vi "Actor Core.vi"(8 "error in":errorcluster, 11 "Test Actor in":refnum<class "Dummy Actor.lvclass">) -> (0 "error out":errorcluster, 3 "Actor out":refnum<class "Actor.lvclass">)   [LabVIEW 2020, in "Test.lvlib" / "Dummy Actor.lvclass"]
doc: "(<B>Filename</B>: Actor Framework.lvlib:Actor.lvclass:Actor Core.vi)\n\nReceives messages to the actor, reacts to them, and initiates any error handling that may shut the actor down.\n\nDescendant classes may override this VI to append parallel tasks for the actor to complete while it handles messages. Overrides use the Call Parent Method node."
uses:
  Dummy Actor.lvclass
  PPL/HDH.Actor Framework.Core.Actor.lvlibp/1abvi3w/vi.lib/ActorFramework/Actor/Actor.lvclass
  PPL/HDH.Actor Framework.Core.File Writer_TDMS.lvlibp/File Writer_TDMS/File Writer_TDMS.lvclass
  PPL/HDH.Actor Framework.Core.Publisher.lvlibp/Publisher Messages/Launch Subscriber Msg/Launch Subscriber Msg.lvclass
  C:/Current projects/WS/PPL/HDH.Actor Framework.Core.Actor.lvlibp/1abvi3w/vi.lib/ActorFramework/Actor/Actor.lvclass
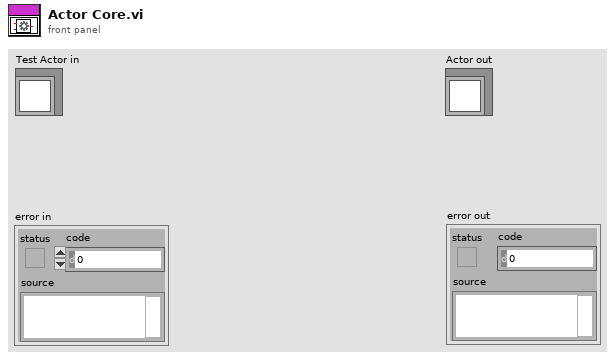
[diagram p1: front panel]
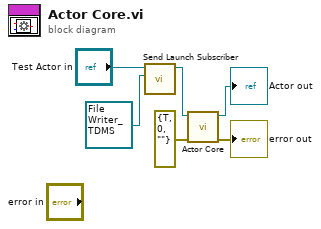
[diagram p0: block diagram]
diagram:
  n1 = call "Send Launch Subscriber.vi"("Actor to Launch"=refnum<class "File Writer_TDMS.lvclass"> refnum ("HDH.Actor Framework.Core.File Writer_TDMS.lvlibp:File Writer_TDMS.lvclass"), "Actor in"="Test Actor in") -> ("Actor out"=w3:refnum<class "Dummy Actor.lvclass">)  [unwired: 7 in, 2 out]
  n2 = call-parent "Actor Core.vi"("error in"=errorcluster {"status"=TRUE, "code"=0, "source"=""}, "Actor in"=w3) -> ("error out"=→"error out":errorcluster, "Actor out"=→"Actor out":refnum<class "Actor.lvclass">)  [unwired: 8 in]
